vi "Main Page.vi"(8 "error in (no error)":errorcluster, 11 "Node Ptr":T3 format="%.0x") -> (0 "error out":errorcluster)   [LabVIEW 2014, in "SLSC configuration System Explorer.lvlib"]
uses:
  SLSC configuration System Explorer.lvlib
  <vilib>/NI Veristand/Custom Device API/Custom Device Item Ref.ctl
  Shared/Type Defs/RIO Device Address.ctl
  Type Defs/Valid.ctl
  Shared/Constants.vi
  <vilib>/NI Veristand/Custom Device API/Get Item Property (U16).vi
  <vilib>/NI Veristand/Custom Device API/Custom Device API.lvlib
  Shared/SLSC configuration Shared.lvlib
  <vilib>/NI Veristand/Custom Device Tools/Custom Device Utility Library/Custom Device Utility Library.lvlib
panel:
  out "Valid?":T1
  out "SLSC SPI Version":string
  out "Custom Device Version":string
  in  "Header 5":cluster{"Section Name":string}={"Section Name"="Slot Configuration"}
  out "Slot Configuration":string[][](table)
  out "SPI Clock Frequency (Hz)":dbl
  in  "Sample Rate (S/s)":u32 min=1 max=40000000
  in  "FPGA Load Delay (s)":u8
  in  "SPI Divide Value":u8 min=1
  in  "Header 4":cluster{"Section Name":string}={"Section Name"="SPI Configuration"}
  in  "Header 3":cluster{"Section Name":string}={"Section Name"="FPGA Configuration"}
  in  "RIO Device Address":T2="RIO0"
  in  "Path":path
  in  "Header":cluster{"Section Name":string}={"Section Name"="SLSC Custom Device Settings"}
  in  "Name":string
  # "120 MHz"
  # "___________________________________"
  # "="
  # "("
  # "+ 1) x 2"
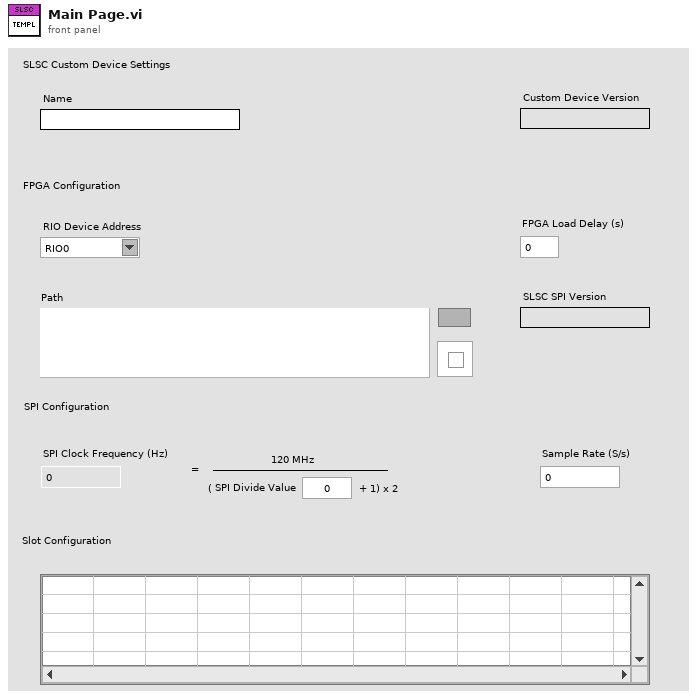
[diagram p1: front panel]
types:
  T1 = typedef "SLSC configuration System Explorer.lvlib/Valid.ctl" = bool
  T2 = typedef "SLSC configuration System Explorer.lvlib/RIO Device Address.ctl" = string
  T3 = typedef "Custom Device API.lvlib/Custom Device Item Ref.ctl" = u64
  T4 = typedef "Custom Device API.lvlib/Custom Device Item Info.ctl" = cluster{"Name":string, "Is Channel":bool, "GUID":string, "Is Waveform":bool}
  T5 = typedef "SLSC configuration System Explorer.lvlib/SLSC Bitfile Info.ctl" = cluster{"FPGA Settings":string, "FIFO Name":string, "Max # of Racks":u8, "UEGO Simulation Names":string[]}
  T6 = typedef "SLSC configuration Shared.lvlib/Card Position.ctl" = cluster{"Rack #":u8, "Slot #":T7}
  T7 = typedef "SLSC configuration Shared.lvlib/Slot #.ctl" = u8
  T8 = typedef "Custom Device API.lvlib/Custom Device Commands.ctl" = enum16{"Default", "Item renamed", "Shutdown", "Dynamic button pressed"}
  T9 = typedef "LVPoint32TypeDef.ctl" = cluster{"Horizontal":i32, "Vertical":i32}
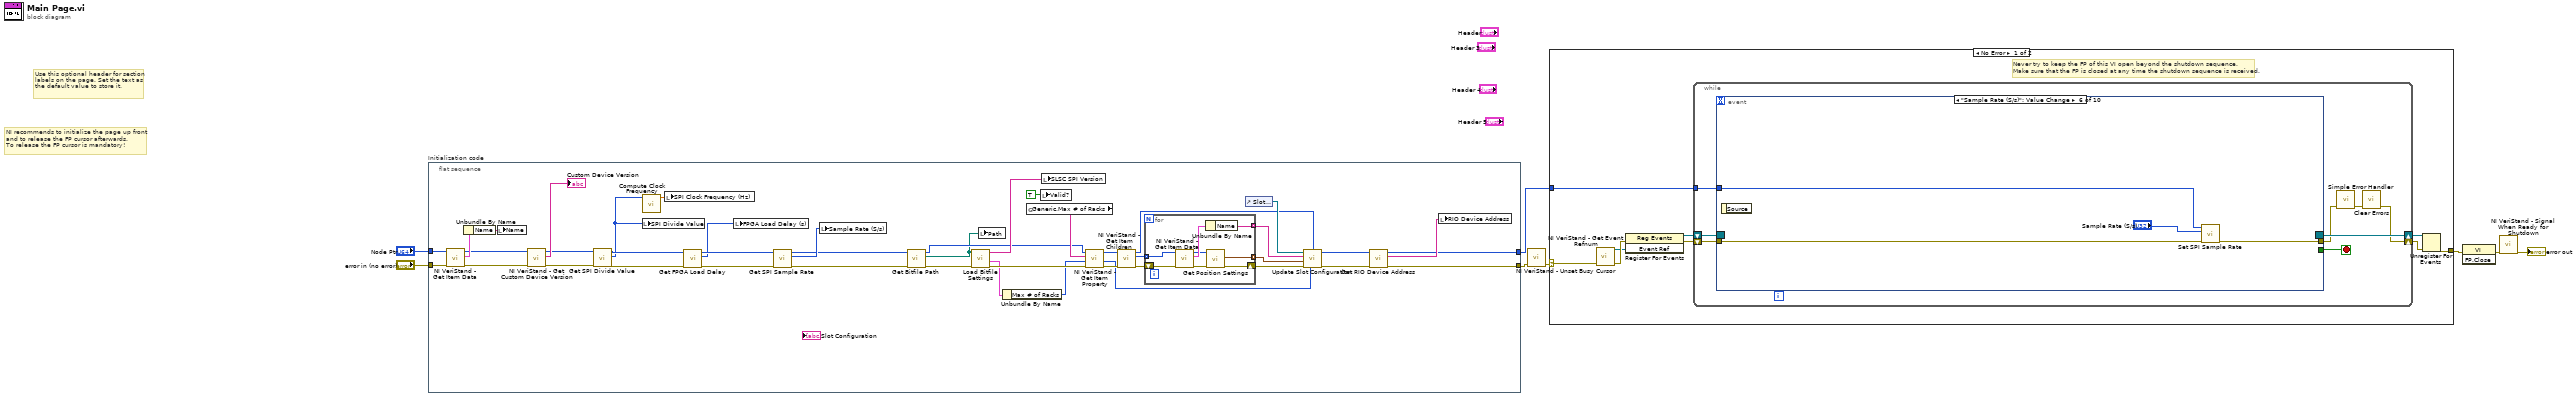
[diagram p0: block diagram]
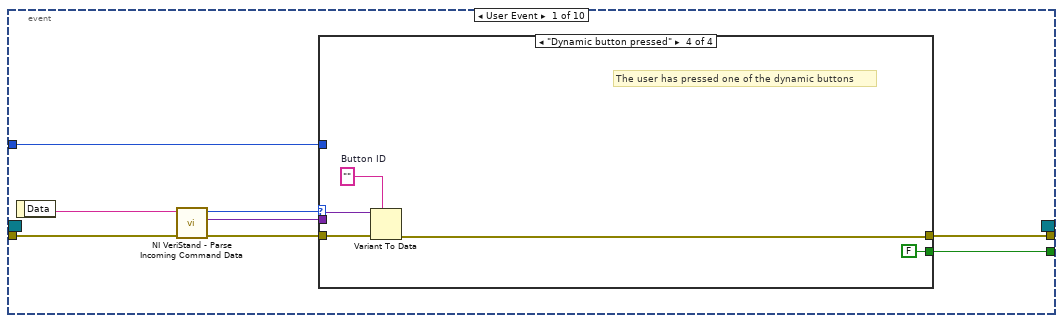
[diagram p2: hidden frame]
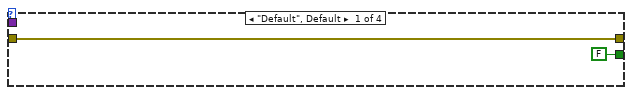
[diagram p3: hidden frame]
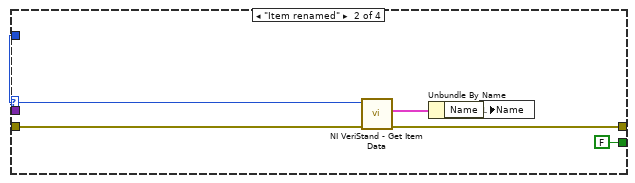
[diagram p4: hidden frame]
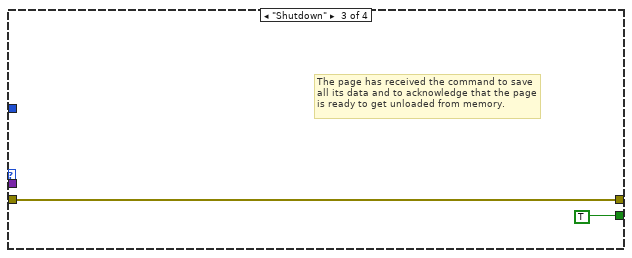
[diagram p5: hidden frame]
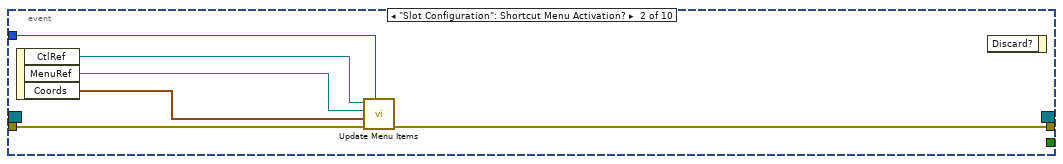
[diagram p6: hidden frame]
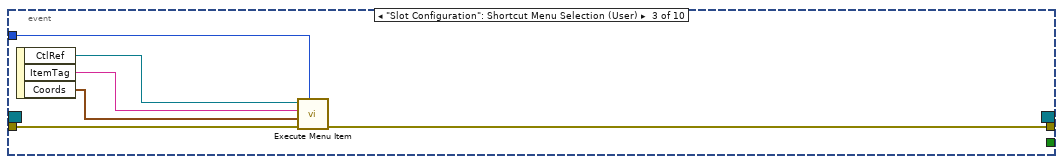
[diagram p7: hidden frame]
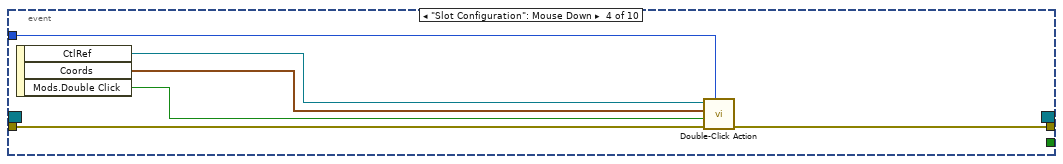
[diagram p8: hidden frame]
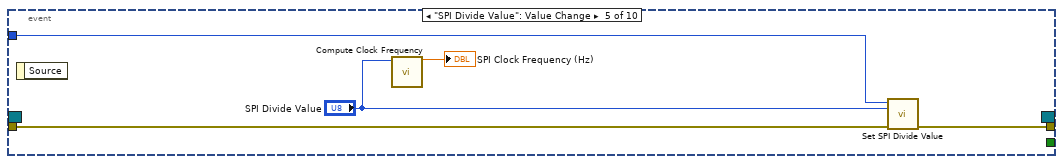
[diagram p9: hidden frame]
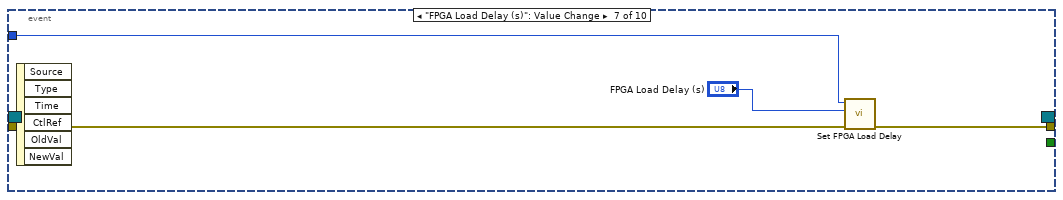
[diagram p10: hidden frame]
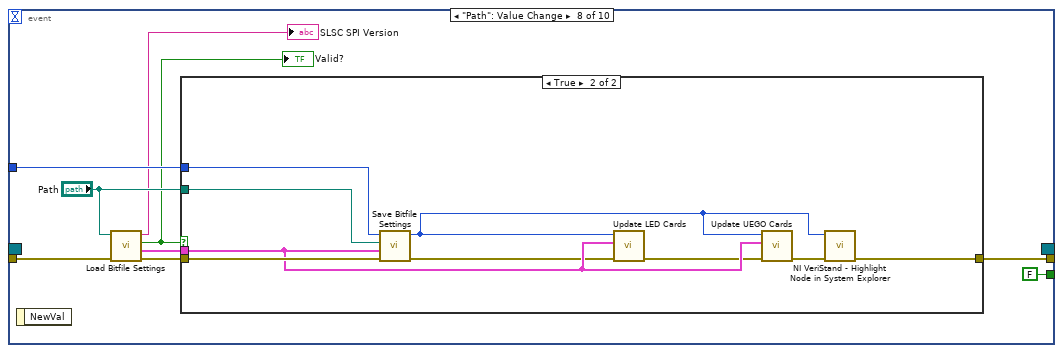
[diagram p11: hidden frame]
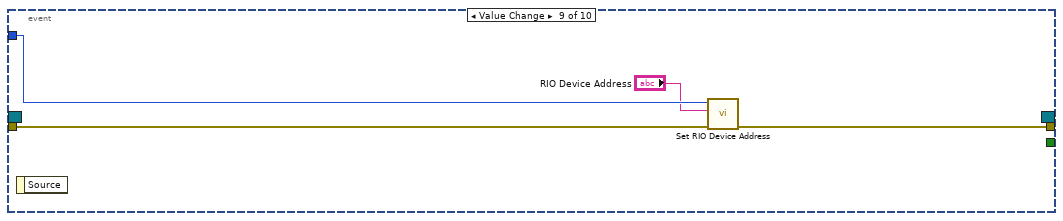
[diagram p13: hidden frame]
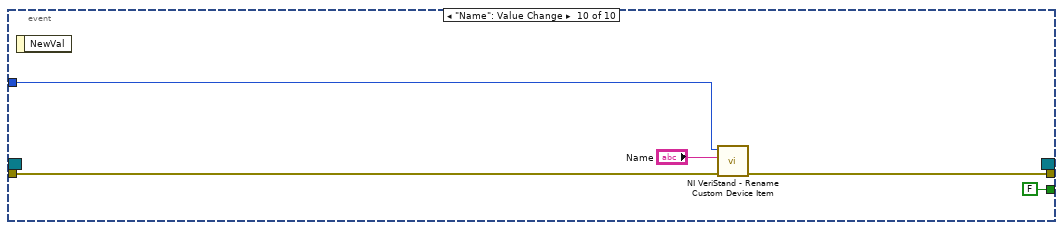
[diagram p14: hidden frame]
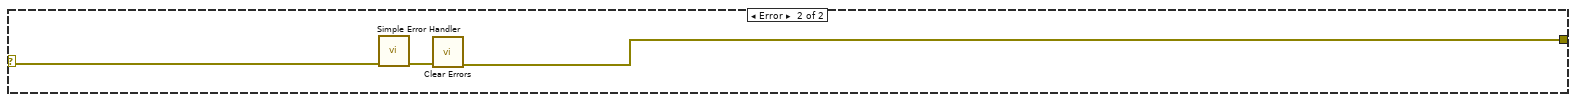
[diagram p15: hidden frame]
diagram:
  # "Use this optional header for section labels on the page. Set the text as the default value to store it."
  # "NI recommends to initialize the page up front\nand to release the FP cursor afterwards.\nTo release the FP cursor is mandatory!"
  n1 = flat-sequence "Initialization code" {
    tunnel: "error in (no error)" -> [w42]
    tunnel: "Node Ptr" -> [w43]
    tunnel: [w44] -> w4
    tunnel: [w15] -> w1
    frame #0 {
      n2 = call <vilib>:"NI VeriStand - Get Item Data.vi"("error in (no error)"=w42, "Item Ref in"=w43) -> ("error out"=w34:errorcluster, "Item Info"=w50:T4, "Item Ref out"=w35:T3)  [unwired: 7 out]
      n3 = Unbundle By Name(w50) -> ("Name"=w49:string)
      n4 = local write "Name"(w49) -> ()
      n5 = call <vilib>:"NI VeriStand - Get Custom Device Version.vi"("error in (no error)"=w34, "Device Ref in"=w35) -> ("error out"=w29:errorcluster, "Value"=→"Custom Device Version":string, "Device Ref out"=w30:T3)  [unwired: 7 in]
      n6 = call "Get SPI Divide Value.vi"("error in (no error)"=w29, "Device Ref in"=w30) -> ("error out"=w47:errorcluster, "SPI Divide Value"=w11:u16, "Item Ref out"=w12:T3)  [unwired: 7 in]
      n7 = call "Compute Clock Frequency.vi"("SPI Divide Value"=w11) -> ("SPI Clock Frequency (Hz)"=w48:dbl)  [unwired: 10 in]
      n8 = local write "SPI Divide Value"(w11) -> ()
      n9 = local write "SPI Clock Frequency (Hz)"(w48) -> ()
      n10 = call "Get FPGA Load Delay.vi"("error in (no error)"=w47, "Item Ref in"=w12) -> ("error out"=w46:errorcluster, "FPGA Load Delay (s)"=w9:u16, "Item Ref out"=w10:T3)  [unwired: 7 in]
      n11 = local write "FPGA Load Delay (s)"(w9) -> ()
      n12 = call "Get SPI Sample Rate.vi"("error in (no error)"=w46, "Item Ref in"=w10) -> ("error out"=w45:errorcluster, "SPI Sample Rate"=w14:u32, "Item Ref out"=w13:T3)  [unwired: 7 in]
      n13 = local write "Sample Rate (S/s)"(w14) -> ()
      n14 = call "Get Bitfile Path.vi"("error in (no error)"=w45, "Item Ref in"=w13) -> ("error out"=w32:errorcluster, "Bitfile Path"=w17:path, "Item Ref out"=w18:T3)  [unwired: 7 in]
      n15 = call "Load Bitfile Settings.vi"("error in (no error)"=w32, "bitfile path"=w17) -> ("error out"=w27:errorcluster, "Bitfile Info"=w19:T5, "SLSC version string"=w31:string)  [unwired: 6 in, 1 out]
      n16 = local write "Path"(w17) -> ()
      n17 = Unbundle By Name(w19) -> ("Max # of Racks"=w26:u8)
      n18 = global read "Constants.vi" "Generic.Max # of Racks"() -> (w28:string)
      n19 = local write "Valid?"(T1 TRUE ("Valid?")) -> ()
      n20 = local write "SLSC SPI Version"(w31) -> ()
      n21 = call-poly <vilib>:"NI VeriStand - Get Item Property.vi"("error in (no error)"=w27, "Default Value"=w26, "Property Name"=w28, "Item Ref in"=w18) -> ("error out"=w25:errorcluster, "Value"=w21:u16, "Item Ref out"=w24:T3)  [unwired: 4 in, 1 out]
      n22 = call <vilib>:"NI VeriStand - Get Item Children.vi"("error in (no error)"=w25, "Item Ref in"=w24) -> ("error out"=w40:errorcluster, "Child Refs"=w41:T3[], "Item Ref out"=w22:T3)  [unwired: 6 in, 1 out]
      n23 = for {
        tunnel: w41 -> [w58] mode=indexing
        shift-right: [w52] -> w39
        shift-left: w40 -> [w57]
        tunnel: [w55] -> w37 mode=indexing
        tunnel: [w51] -> w36 mode=indexing
        n24 = call <vilib>:"NI VeriStand - Get Item Data.vi"("error in (no error)"=w57, "Item Ref in"=w58) -> ("error out"=w54:errorcluster, "Item Info"=w56:T4, "Item Ref out"=w53:T3)  [unwired: 7 out]
        n25 = Unbundle By Name(w56) -> ("Name"=w55:string)
        n26 = call "Get Position Settings.vi"("error in (no error)"=w54, "Item Ref in"=w53) -> ("error out"=w52:errorcluster, "Card Position"=w51:T6)  [unwired: 7 in, 1 out]
      }
      n27 = control-ref of="Slot Configuration"() -> (w38:refnum<vi>)
      n28 = call "Update Slot Configuration.vi"("Max # of Racks"=w21, "error in (no error)"=w39, "Card Position"=w36, "Card Name"=w37, "Slot Configuration in"=w38) -> ("error out"=w23:errorcluster)  [unwired: 5 in, 1 out]
      n29 = call "Get RIO Device Address.vi"("error in (no error)"=w23, "Item Ref in"=w22) -> ("error out"=w44:errorcluster, "RIO Device Address"=w16:string, "Item Ref out"=w15:T3)  [unwired: 7 in]
      n30 = local write "RIO Device Address"(w16) -> ()
    }
  }
  n31 = call <vilib>:"NI VeriStand - Unset Busy Cursor.vi"("error in (no error)"=w4) -> ("error out"=w3:errorcluster)  [unwired: 10 out]
  n32 = case shown="No Error" w3 {
    selector: w3 -> [w59 w160]
    tunnel: [w64 w158] -> w8
    tunnel: w1 -> [w60 _]
    frame No Error {
      # "Never try to keep the FP of this VI open beyond the shutdown sequence.\nMake sure that the FP is closed at any time the shutdown sequence is received."
      n33 = call <vilib>:"NI VeriStand - Get Event Refnum.vi"("error in (no error)"=w59) -> ("error out"=w67:errorcluster, "Event Ref"=w63:refnum<user-event>)  [unwired: 9 out]
      n34 = register-events(error in=w67, w63) -> (reference out=w61:refnum<event-registration>, error out=w62:errorcluster)  [unwired: 1 in]
      n35 = while {
        tunnel: w60 -> [w71]
        shift-right: [w68] -> w65
        shift-left: w62 -> [w74]
        shift-right: [w75] -> w66
        shift-left: w61 -> [w73]
        stop <- w72 stop-if-true
        n36 = event shown="[5] \"Sample Rate (S/s)\": Value Change" {
          selector: w73 -> [_ _ _ _ _ _ _ _ _ _]
          dyn-events: [_ _ _ _ _ _ _ _ _ _] -> w75
          timeout: _ -> [_ _ _ _ _ _ _ _ _ _]
          tunnel: w74 -> [w83 w102 w110 w116 w120 w125 w129 w135 w152 w157]
          tunnel: [w79 _ _ _ _ _ _ FALSE _ FALSE] -> w72
          tunnel: [w78 w101 w105 w111 w119 w124 w128 w137 w151 w156] -> w70
          tunnel: w71 -> [w77 w99 w106 w112 w121 w123 w127 w138 w150 w155]
          event User Event {
            n37 = event-data() -> ("Data"=w82:string)  [unwired: 1 out]
            n38 = call <vilib>:"NI VeriStand - Parse Incoming Command Data.vi"("error in (no error)"=w83, "Incoming data"=w82) -> ("error out"=w81:errorcluster, "Outgoing data"=w76:variant, "Action"=w80:T8)  [unwired: 7 out]
            n39 = case shown="\"Dynamic button pressed\"" w80 {
              tunnel: w81 -> [w85 w91 w92 w98]
              tunnel: [FALSE FALSE TRUE FALSE] -> w79
              tunnel: [w85 w88 w92 w95] -> w78
              tunnel: w77 -> [_ w90 _ _]
              tunnel: w76 -> [_ _ _ w97]
              frame "Default", Default {
              }
              frame "Item renamed" {
                n40 = call <vilib>:"NI VeriStand - Get Item Data.vi"("error in (no error)"=w91, "Item Ref in"=w90) -> ("error out"=w88:errorcluster, "Item Info"=w89:T4)  [unwired: 8 out]
                n41 = Unbundle By Name(w89) -> ("Name"=w87:string)
                n42 = local write "Name"(w87) -> ()
              }
              frame "Shutdown" {
                # "The page has received the command to save all its data and to acknowledge that the page is ready to get unloaded from memory."
              }
              frame "Dynamic button pressed" {
                w96 = ""  # Button ID
                # "The user has pressed one of the dynamic buttons"
                n43 = Variant To Data(error in=w98, type=w96, Variant=w97) -> (error out=w95:errorcluster)  [unwired: 1 out]
              }
            }
          }
          event "Slot Configuration": Shortcut Menu Activation? {
            n44 = event-data() -> ("CtlRef"=w104:refnum<vi>, "MenuRef"=w100:refnum<k9>, "Coords"=w103:T9)  [unwired: 1 out]
            n45 = call "Update Menu Items.vi"("Device Ref in"=w99, "error in (no error)"=w102, "Coords"=w103, "MenuRef"=w100, "Table in"=w104) -> ("error out"=w101:errorcluster)  [unwired: 6 in]
            n46 = event-data() -> ()  [unwired: 2 in, 1 out]
          }
          event "Slot Configuration": Shortcut Menu Selection (User) {
            n47 = event-data() -> ("CtlRef"=w107:refnum<vi>, "ItemTag"=w108:string, "Coords"=w109:T9)  [unwired: 1 out]
            n48 = call "Execute Menu Item.vi"("Device Ref in"=w106, "error in (no error)"=w110, "Coords"=w109, "ItemTag"=w108, "CtlRef"=w107) -> ("error out"=w105:errorcluster)  [unwired: 6 in]
          }
          event "Slot Configuration": Mouse Down {
            n49 = event-data() -> ("CtlRef"=w113:refnum<vi>, "Coords"=w114:T9, "Mods.Double Click"=w115:bool)  [unwired: 1 out]
            n50 = call "Double-Click Action.vi"("Device Ref in"=w112, "error in (no error)"=w116, "Mods.Double Click"=w115, "Coords"=w114, "CtlRef"=w113) -> ("error out"=w111:errorcluster)  [unwired: 6 in]
          }
          event "SPI Divide Value": Value Change {
            n51 = event-data() -> ()  [unwired: 2 out]
            n52 = call "Compute Clock Frequency.vi"("SPI Divide Value"="SPI Divide Value") -> ("SPI Clock Frequency (Hz)"=→"SPI Clock Frequency (Hz)":dbl)  [unwired: 10 in]
            n53 = call "Set SPI Divide Value.vi"("error in (no error)"=w120, "SPI Divide Value"="SPI Divide Value", "Item Ref in"=w121) -> ("error out"=w119:errorcluster)  [unwired: 7 in, 1 out]
          }
          event "Sample Rate (S/s)": Value Change {
            n54 = event-data() -> ()  [unwired: 2 out]
            n55 = call "Set SPI Sample Rate.vi"("error in (no error)"=w125, "Sample Rate (S/s)"="Sample Rate (S/s)", "Item Ref in"=w123) -> ("error out"=w124:errorcluster)  [unwired: 7 in, 1 out]
          }
          event "FPGA Load Delay (s)": Value Change {
            n56 = event-data() -> ()  [unwired: 7 out]
            n57 = call "Set FPGA Load Delay.vi"("error in (no error)"=w129, "FPGA Load Delay (s)"="FPGA Load Delay (s)", "Item Ref in"=w127) -> ("error out"=w128:errorcluster)  [unwired: 7 in, 1 out]
          }
          event "Path": Value Change {
            n58 = event-data() -> ()  [unwired: 2 out]
            n59 = call "Load Bitfile Settings.vi"("error in (no error)"=w135, "bitfile path"="Path") -> ("error out"=w133:errorcluster, "Bitfile Info"=w131:T5, "Valid?"=w130:bool, "SLSC version string"=→"SLSC SPI Version":string)  [unwired: 6 in]
            "Valid?" <- w130
            n60 = case shown="True" w130 {
              tunnel: w138 -> [_ w147]
              tunnel: [w139 w144] -> w137
              tunnel: "Path" -> [_ w146]
              tunnel: w133 -> [w139 w148]
              tunnel: w131 -> [_ w143]
              frame False {
              }
              frame True {
                n61 = call "Save Bitfile Settings.vi"("error in (no error)"=w148, "Bitfile Info"=w143, "Path"=w146, "Device Ref in"=w147) -> ("error out"=w141:errorcluster, "Device Ref out"=w142:T3)  [unwired: 6 in]
                n62 = call "Update LED Cards.vi"("error in (no error)"=w141, "Bitfile Info"=w143, "Device Ref in"=w142) -> ("error out"=w140:errorcluster)  [unwired: 8 in]
                n63 = call "Update UEGO Cards.vi"("error in (no error)"=w140, "Bitfile Info"=w143, "Device Ref in"=w142) -> ("error out"=w145:errorcluster)  [unwired: 8 in]
                n64 = call <vilib>:"NI VeriStand - Highlight Node in System Explorer.vi"("error in (no error)"=w145, "Item Ref in"=w142) -> ("error out"=w144:errorcluster)  [unwired: 8 in, 1 out]
              }
            }
          }
          event Value Change {
            n65 = event-data() -> ()  [unwired: 2 out]
            n66 = call "Set RIO Device Address.vi"("error in (no error)"=w152, "RIO Device Address"="RIO Device Address", "Item Ref in"=w150) -> ("error out"=w151:errorcluster)  [unwired: 7 in, 1 out]
          }
          event "Name": Value Change {
            n67 = event-data() -> ()  [unwired: 2 out]
            n68 = call <vilib>:"NI VeriStand - Rename Custom Device Item.vi"("error in (no error)"=w157, "New Name"="Name", "Item Ref in"=w155) -> ("error out"=w156:errorcluster)  [unwired: 1 in, 7 out]
          }
        }
        n69 = call <vilib>:"Simple Error Handler.vi"("error in (no error)"=w70) -> ("error out"=w69:errorcluster)  [unwired: 1 in, 7 out]
        n70 = call <vilib>:"Clear Errors.vi"("error in (no error)"=w69) -> ("error out"=w68:errorcluster)  [unwired: 1 in, 5 out]
      }
      n71 = Unregister For Events(event registration refnum=w66, error in=w65) -> (error out=w64:errorcluster)
    }
    frame Error {
      n72 = call <vilib>:"Simple Error Handler.vi"("error in (no error)"=w160) -> ("error out"=w159:errorcluster)  [unwired: 1 in, 7 out]
      n73 = call <vilib>:"Clear Errors.vi"("error in (no error)"=w159) -> ("error out"=w158:errorcluster)  [unwired: 1 in, 5 out]
    }
  }
  n74 = invoke class="VI" method="FP.Close"(error in=w8) -> (error out=w7:errorcluster)  [unwired: 2 in, 2 out]
  n75 = call <vilib>:"NI VeriStand - Signal When Ready for Shutdown.vi"("error in (no error)"=w7) -> ("error out"=→"error out":errorcluster)  [unwired: 10 out]
